vi "Nachtmessung_Temperatur.vi"() -> ()   [LabVIEW 2010]
panel:
  out "error out":errorcluster
  in  "error in":errorcluster
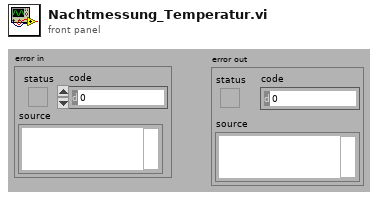
[diagram p1: front panel]
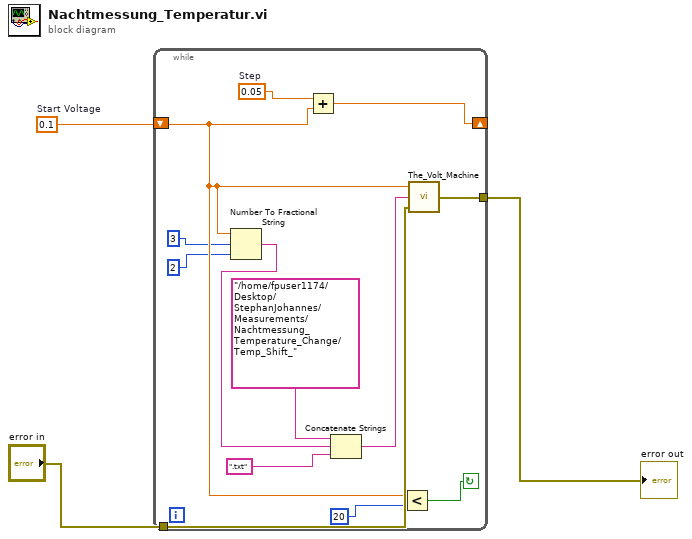
[diagram p0: block diagram]
diagram:
  w3 = 0.1  # Start Voltage
  n1 = while {
    shift-right: [w15] -> _
    shift-left: w3 -> [w10]
    tunnel: "error in" -> [w14]
    tunnel: [w11] -> w1
    stop <- w12 continue-if-true
    w16 = 0.05  # Step
    n2 = Number To Fractional String(number=w10, width (-)=3, precision (6)=2) -> (F-format string=w9:string)  [unwired: 1 in]
    n3 = Add(x=w16, y=w10) -> (x+y=w15:dbl)
    n4 = Concatenate Strings("/home/fpuser1174/Desktop/StephanJohannes/Measurements/Nachtmessung_Temperature_Change/Temp_Shift_", w9, ".txt") -> (w5:string)
    n5 = Less?(x=w10, y=20) -> (x < y?=w12:bool)
    n6 = call "The_Volt_Machine.vi"("error in"=w14, "Adress"=w5, "Voltage"=w10) -> ("error out"=w11:errorcluster)
  }
  "error out" <- w1
